vi "Dashboard Main.vi"() -> ()   [LabVIEW 2017]
uses:
  <vilib>/Utility/miscctls.llb/LVRowAndColumnTypeDef.ctl
  <vilib>/event_ctls.llb/eventvkey.ctl
  <vilib>/Rock Robotics/WPI/Dashboard/WPI_DashboardLogging Global.vi
panel:
  in  "Camera Settings Right":T1={"Frame Rate"=30, "Compression"=30, "Size"=1, "DB Camera Config"=FALSE} {"Frame Rate" scale=1.0..30.0; "Compression" scale=100.0..-1.0; "Size" items=["640x480", "320x240", "160x120"]}
  in  "Camera Name Right":string(combo)="No Camera Selection"
  out "Camera Info":cluster{"Mbps LED":bool, "Mbps":dbl, "fps":dbl} {"fps" format="%#.1g"; "Mbps" format="%#.1g"}
  in  "Camera Settings":T1={"Frame Rate"=30, "Compression"=30, "Size"=1, "DB Camera Config"=FALSE} {"Frame Rate" scale=1.0..30.0; "Compression" scale=100.0..-1.0; "Size" items=["640x480", "320x240", "160x120"]}
  in  "TCP":refnum<k5>
  in  "Rec Mode":enum32{"Stop", "Record", "Playback"}(radio)
  out "Robot IP":string
  out "Image Message":string="Timeout in Camera Communications"
  in  "Dashboard Tab":T2(tab)
  out "PowerCube Loaded":bool
  in  "Si Right":bool
  in  "Select Auto":string(combo)="Select Autonomous ..."
  out "NT Connection":bool
  out "Gyro":dbl(knob) scale=0.0..360.0
  out "Mode":T3(ring)=enum."Auto Disabled"
  out "Boolean":bool
  out "Boolean 2":bool
  out "Boolean 3":bool
  out "Boolean 4":bool
  out "Boolean 5":bool
  out "Boolean 6":bool
  out "Camera Image Right":T4(plugin-control)
  in  "DB/String 9":string
  in  "DB/String 8":string
  in  "DB/String 7":string
  in  "DB/String 6":string
  in  "DB/String 5":string
  in  "DB/String 4":string
  in  "DB/String 3":string
  in  "DB/String 2":string
  in  "DB/String 1":string
  in  "DB/String 0":string
  in  "DB/Slider 0":dbl(slide) scale=0.0..5.0
  in  "DB/Slider 1":dbl(slide) scale=0.0..5.0
  in  "DB/Slider 2":dbl(slide) scale=0.0..5.0
  in  "DB/Slider 3":dbl(slide) scale=0.0..5.0
  out "DB/LED 3":bool
  out "DB/LED 2":bool
  out "DB/LED 1":bool
  out "DB/LED 0":bool
  in  "DB/Button 3":bool
  in  "DB/Button 2":bool
  in  "DB/Button 1":bool
  in  "DB/Button 0":bool caption="New Name"
  out "Alliance":string
  out "GameData":string
  in  "Test Slider":dbl(slide) scale=0.0..100.0 scale format="%#_3g"
  in  "On/Off":bool caption="Solenoid"
  in  "Test Name":u16(ring) items=["Select the test to run..."]
  in  "Test Tree":string(tree)
  in  "Motor":cluster{"Value":dbl, "Enable":bool} {"Value" scale=-1.0..1.0 scale format="%#_3g"}
  out "Progress":T5 {"Test Progress" scale=0.0..100.0}
  in  "Rev/Fwd":cluster{"Forward":bool, "Reverse":bool}
  in  "Test Ring":u16(ring) items=["Monochrome", "Color"]
  out "Cmd Status":string
  in  "Execute Command":bool
  in  "Command Params":string[][](table)
  in  "Command Selection":i32(listbox)
  in  "CheckList":i32(listbox)
  out "Tree":string(tree)
  out "Camera Image":T4(plugin-control)
  out "Background":bool
  in  "Camera Name":string(combo)="No Camera Selection"
  # "HW"
  # "HW"
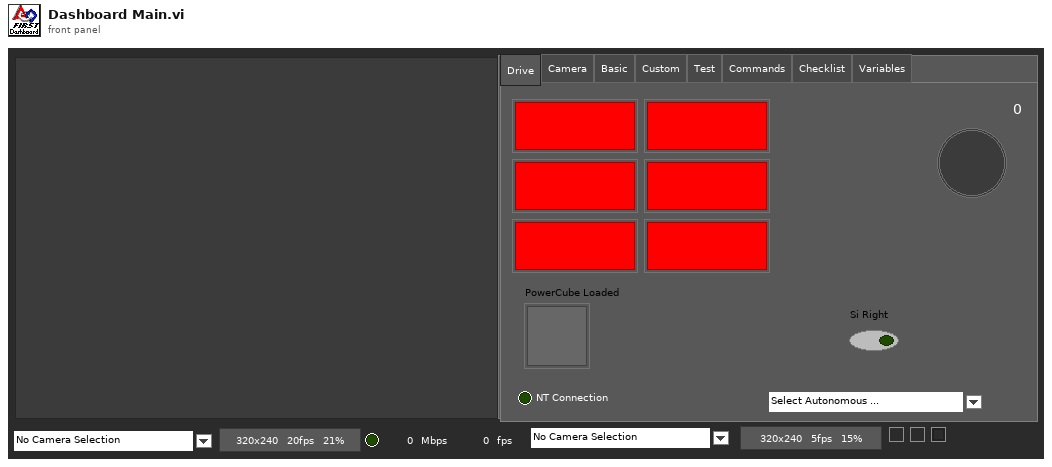
[diagram p1: front panel]
types:
  T1 = cluster{"Frame Rate":i32, "Compression":i32, "Size":u16, "DB Camera Config":bool}
  T2 = enum32{"Drive", "Camera", "Basic", "Custom", "Test", "Commands", "Checklist", "Variables"}
  T3 = enum8{"Tele-Op Disabled", "Tele-Op Enabled", "Auto Disabled", "Auto Enabled", "Test Disabled", "Test Enabled", "Disconnected", "No Code", "E-Stop"}
  T4 = typedef "IMAQ Image.ctl" = refnum<image>
  T5 = cluster{"Test Progress":u8, "Test Progress Text":string}
  T6 = cluster{"Save Path":path, "Interval (s)":dbl, "Keep":i32}
  T7 = typedef "Image Type" = u32
  T8 = cluster{"IDs":cluster{"RPC field ID":u16, "Unique ID":u16}, "String":string}
  T9 = cluster{"Error Strings":string, "Disable Counts":cluster{u16, u16}, "Rail Faults":cluster{u16, u16, u16}, "Robot IP":string, "DB Mode":u8, "Event Info":cluster{"Name":string, "Type":u8, "Number":u16, "Replay":u8}}
  T10 = cluster{"Storage":cluster{"Disk Free":u64, "RAM Block":u32, "RAM free":u32}, "CPU Utilization":cluster{"CPU % ISR":sgl, "CPU % Time Crit":sgl, "CPU % Timed Str":sgl, "CPU % High":sgl, "CPU % Above":sgl, "CPU % Normal":sgl, "CPU % Low":sgl}, "CAN":cluster{"% Bus Utilization":sgl, "Bus Off Cnt":u32, "TX_FIFO Full Cnt":u32, "Receive Error Cnt":u8, "Transmit Error Cnt":u8}, "HID":cluster{"HID Outputs":u32, "Rumble Low":u16, "Rumble High":u16}[]}
  T11 = cluster{"Status bits":cluster{"Test Mode":bool, "Autonomous":bool, "Enabled":bool, "Code Start":bool, "Brownout":bool, "Reserved 2":bool, "Reserved 3":bool, "E-Stop":bool}, "Code Trace":cluster{"Disabled":bool, "TeleOp":bool, "Auto":bool, "Test":bool}, "Controller Type":enum16{"unknown", "cRIO", "roboRio"}, "Code?":enum16{"unknown", "noCode", "code"}, "Battery V":dbl}
  T12 = cluster{"Control Bits":cluster{"TestMode":bool, "Autonomous":bool, "Enabled":bool, "FMS Present":bool, bool, bool, bool, "E-Stop":bool}, "Team Station ":u8, "Countdown":sgl, "Joystick Values":cluster{"Axes":dbl[], "Buttons":bool[], "POVs":i16[]}[]}
  T13 = cluster{"Axes":dbl[], "Buttons":bool[], "POVs":i16[]}[]
  T14 = cluster{"Axes":dbl[], "Buttons":bool[], "POVs":i16[]}
  T15 = cluster{"Camera Image":refnum<vi>, "Dashboard Tab":refnum<vi>, "Background":refnum<vi>, "Rec Mode":refnum<vi>, "Test Slider":refnum<vi>, "On/Off ":refnum<vi>, "Test Ring":refnum<vi>, "Rev/Fwd":refnum<vi>, "Test Name":refnum<vi>, "Motor":refnum<vi>, "Progress":refnum<vi>, "CheckList":refnum<vi>, "Tree":refnum<vi>, "Test Tree":refnum<vi>, "Command Params":refnum<vi>, "Command Selection":refnum<vi>, "Execute Command":refnum<vi>, "Cmd Status":refnum<vi>, "Camera Settings":refnum<vi>, "Camera Name":refnum<vi>, "Camera Info":refnum<vi>, "Camera Settings Right":refnum<vi>, "Camera Name Right":refnum<vi>, "Camera Image Right":refnum<vi>}
  T16 = cluster{"Camera Name":string, string, "Saved DB Images Info":cluster{"Save Path":path, "Interval (s)":dbl, "Keep":i32}}
  T17 = cluster{"Camera Name Right":string, string, "Saved DB Images Info":cluster{"Save Path":path, "Interval (s)":dbl, "Keep":i32}}
  T18 = cluster{"Operation":enum16{"Update", "Clear"}, "Color Box":u32}[]
  T19 = typedef "eventvkey.ctl" = enum16{"ASCII", "Enter", "Return", "Shift", "Ctrl", "Alt", "Cmd", "Opt", "Caps", "NumLock", "Clear", "Break", "Up", "Down", "Left", "Right", "Insert", "Delete", "Home", "End", "PageUp", "PageDown", "Escape", "Help", "Pause", "ScrollLock", "F1", "F2", "F3", "F4", "F5", "F6", "F7", "F8", "F9", "F10", "F11", "F12", "F13", "F14", "F15", "F16", "F17", "F18", "F19", "F20", "F21", "F22", "F23", "F24", "Play", "VolumeUp", "VolumeDown", "Mute", "Two Byte Char"}
  T20 = cluster{"Image Size":bool, "Image Type":bool, "Pixel Value":bool, "ROI Information":bool, "Zoom Factor":bool}
  T21 = cluster{"Operation":enum16{"Update", "Clear"}, "Color Box":u32}
  T22 = typedef "LVRowAndColumnTypeDef.ctl" = cluster{"Row":i32, "Column":i32}
  T23 = cluster{"Shift":bool, "Ctrl":bool, "Alt":bool, "Cmd":bool, "Opt":bool}
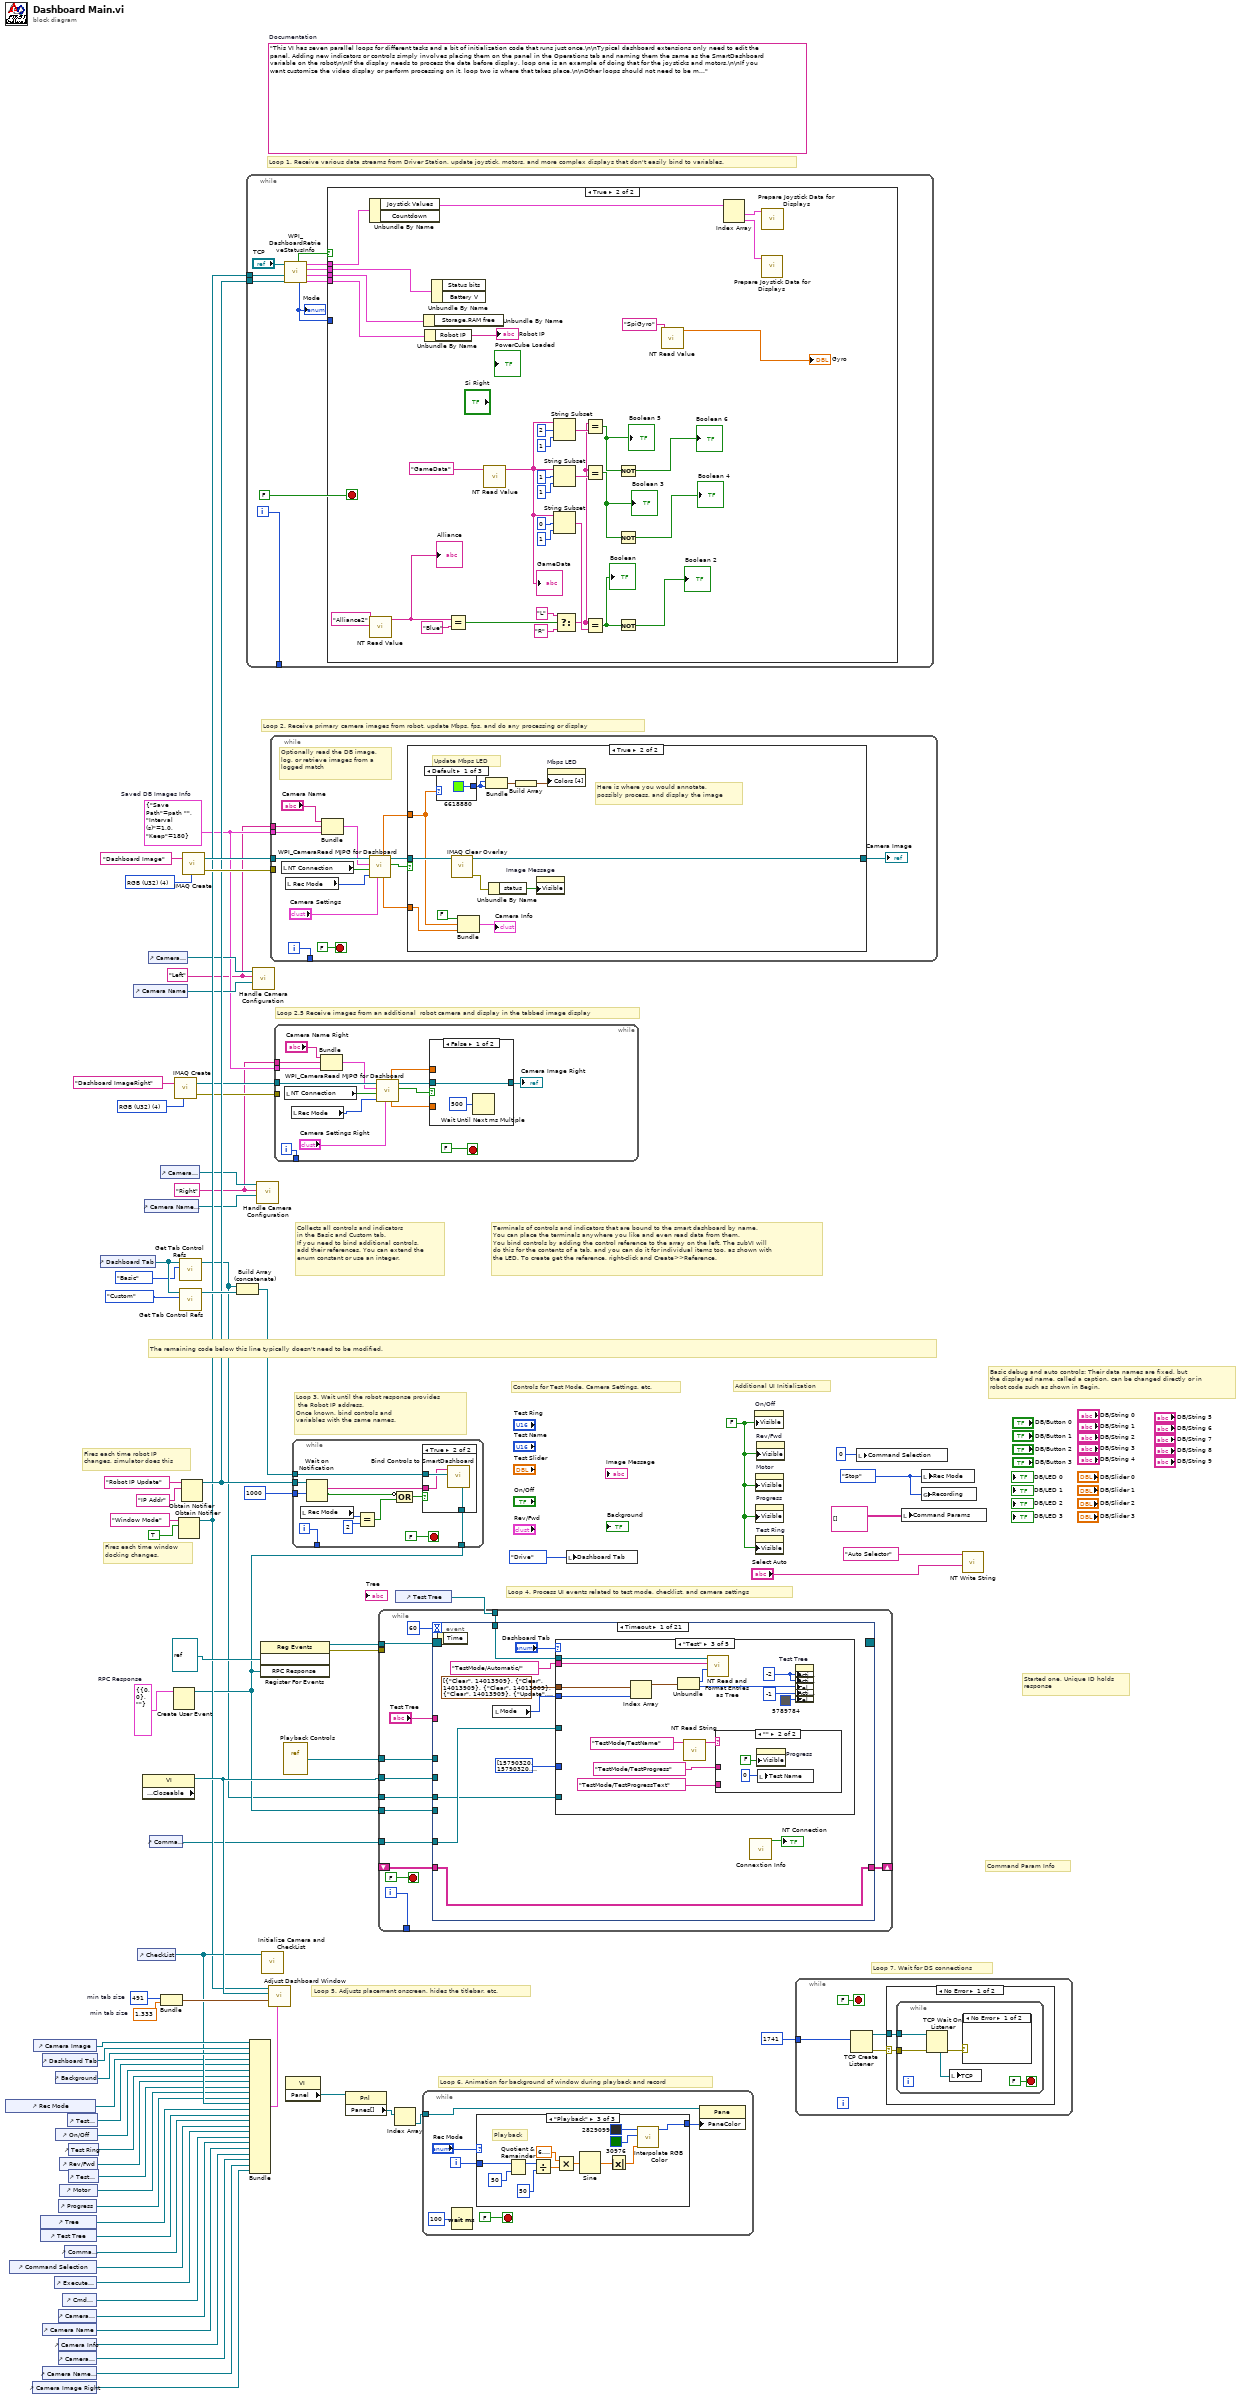
[diagram p0: block diagram]
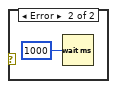
[diagram p3: hidden frame]
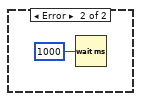
[diagram p4: hidden frame]
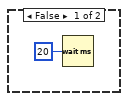
[diagram p5: hidden frame]
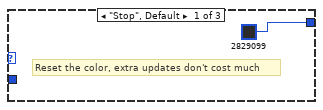
[diagram p6: hidden frame]
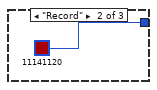
[diagram p7: hidden frame]
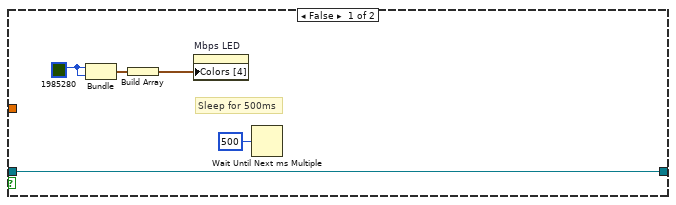
[diagram p9: hidden frame]
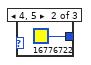
[diagram p10: hidden frame]
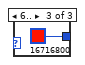
[diagram p11: hidden frame]
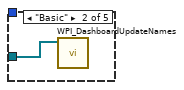
[diagram p13: hidden frame]
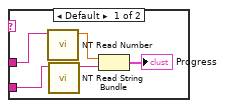
[diagram p14: hidden frame]
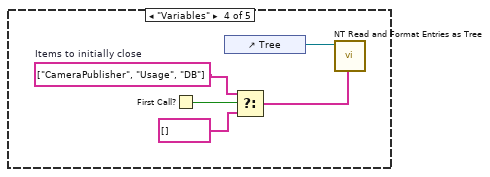
[diagram p15: hidden frame]
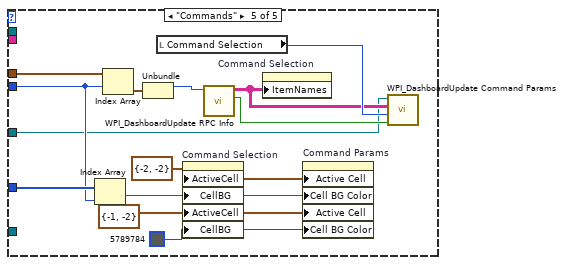
[diagram p16: hidden frame]
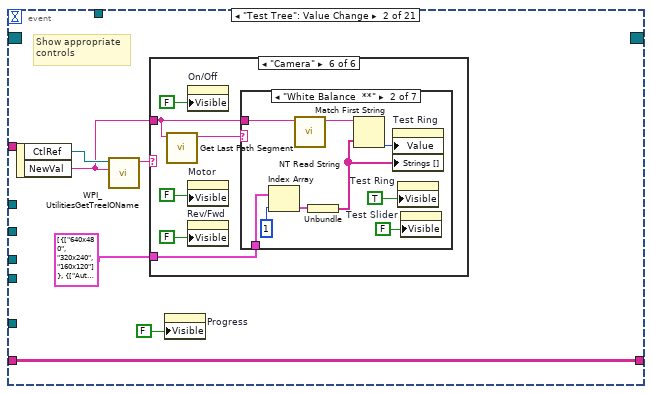
[diagram p17: hidden frame]
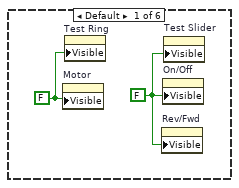
[diagram p18: hidden frame]
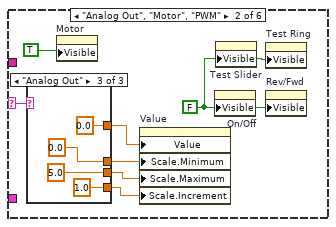
[diagram p19: hidden frame]
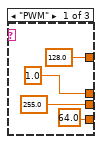
[diagram p20: hidden frame]
diagram:
  w3 = T6 {"Save Path"=path "", "Interval (s)"=1.0, "Keep"=180}  # Saved DB Images Info
  w2 = "Right"
  w1 = "Left"
  w13 = T7 4 items=["Grayscale (U8)", "Grayscale (I16)", "Grayscale (SGL)", "Complex (CSG)", "RGB (U32)", "HSL (U32)", "RGB (U64)"] ("Image Type")
  w29 = T8 {"IDs"={"RPC field ID"=0, "Unique ID"=0}, "String"=""}  # RPC Response
  w52 = 491  # min tab size
  w51 = 1.333  # min tab size
  w59 = enum32{"Stop", "Record", "Playback"}."Stop" ("Rec Mode")
  w36 = FALSE ("Visible")
  (unwired) "This VI has seven parallel loops for different tasks and a bit of initialization code that runs just once.\n\nTypical dashboard extensions only need to edit the panel. Adding new indicators or controls simply involves placing them on the panel in the Operations tab and naming them the same as the SmartDashboard variable on the robot\n\nIf the display needs to process the data before display, loop one is an example of doing that for the joysticks and motors.\n\nIf you want customize the video display or perform processing on it, loop two is where that takes place.\n\nOther loops should not need to be modified. They are pretty standard, and document the task they perform."  # Documentation
  w76 = T7 4 items=["Grayscale (U8)", "Grayscale (I16)", "Grayscale (SGL)", "Complex (CSG)", "RGB (U32)", "HSL (U32)", "RGB (U64)"] ("Image Type")
  # "Loop 2.5 Receive images from an additional  robot camera and display in the tabbed image display"
  # "Command Param Info"
  # "Started one, Unique ID holds\nresponse"
  # "Loop 7. Wait for DS connections"
  # "Basic debug and auto controls: Their data names are fixed, but\nthe displayed name, called a caption, can be changed directly or in\nrobot code such as shown in Begin."
  # "Controls for Test Mode, Camera Settings, etc."
  # "Additional UI Initialization"
  # "Loop 6. Animation for background of window during playback and record"
  # "Fires each time robot IP\nchanges, simulator does this"
  # "Fires each time window\ndocking changes."
  # "Collects all controls and indicators\nin the Basic and Custom tab.\nIf you need to bind additional controls,\nadd their references. You can extend the\nenum constant or use an integer."
  # "The remaining code below this line typically doesn't need to be modified."
  # "Loop 4. Process UI events related to test mode, checklist, and camera settings"
  # "Terminals of controls and indicators that are bound to the smart dashboard by name.\nYou can place the terminals anywhere you like and even read data from them.\nYou bind controls by adding the control reference to the array on the left. The subVI will\ndo this for the contents of a tab, and you can do it for individual items too, as shown with\nthe LED. To create get the reference, right-click and Create>>Reference."
  # "Loop 3. Wait until the robot response provides\n the Robot IP address.\nOnce known, bind controls and\nvariables with the same names."
  # "Loop 5. Adjusts placement onscreen, hides the titlebar, etc."
  # "Loop 1. Receive various data streams from Driver Station, update joystick, motors, and more complex displays that don't easily bind to variables."
  # "Loop 2. Receive primary camera images from robot, update Mbps, fps, and do any processing or display"
  n1 = control-ref of="Rec Mode"() -> (w42:refnum<vi>)
  n2 = control-ref of="Command Selection"() -> (w28:refnum<vi>)
  n3 = control-ref of="Camera Image Right"() -> (w6:refnum<vi>)
  n4 = control-ref of="Camera Image"() -> (w54:refnum<vi>)
  n5 = control-ref of="Tree"() -> (w46:refnum<vi>)
  n6 = control-ref of="Test Tree"() -> (w45:refnum<vi>)
  n7 = control-ref of="Dashboard Tab"() -> (w53:refnum<vi>)
  n8 = control-ref of="Camera Name"() -> (w19:refnum<vi>)
  n9 = control-ref of="Camera Name Right"() -> (w7:refnum<vi>)
  n10 = control-ref of="Execute Command"() -> (w30:refnum<vi>)
  n11 = control-ref of="Background"() -> (w49:refnum<vi>)
  n12 = control-ref of="On/Off"() -> (w40:refnum<vi>)
  n13 = control-ref of="Progress"() -> (w37:refnum<vi>)
  n14 = control-ref of="Camera Settings"() -> (w20:refnum<vi>)
  n15 = control-ref of="Camera Info"() -> (w18:refnum<vi>)
  n16 = control-ref of="Camera Settings Right"() -> (w8:refnum<vi>)
  n17 = control-ref of="Rev/Fwd"() -> (w38:refnum<vi>)
  n18 = control-ref of="Motor"() -> (w43:refnum<vi>)
  n19 = control-ref of="Cmd Status"() -> (w24:refnum<vi>)
  n20 = control-ref of="Command Params"() -> (w31:refnum<vi>)
  n21 = control-ref of="Test Slider"() -> (w41:refnum<vi>)
  n22 = control-ref of="Test Ring"() -> (w39:refnum<vi>)
  n23 = control-ref of="Test Name"() -> (w44:refnum<vi>)
  n24 = control-ref of="Dashboard Tab"() -> (w57:refnum<vi>)
  n25 = control-ref of="Camera Name"() -> (w21:refnum<vi>)
  n26 = control-ref of="CheckList"() -> (w47:refnum<vi>)
  n27 = property class="VI" props=["Front Panel.Closeable"]() -> (reference out=w58:refnum<vi>)  [unwired: 2 in, 2 out]
  n28 = control-ref of="Camera Name Right"() -> (w9:refnum<vi>)
  n29 = control-ref of="Camera Settings"() -> (w22:refnum<vi>)
  n30 = control-ref of="Command Params"() -> (w23:refnum<vi>)
  n31 = control-ref of="Camera Settings Right"() -> (w10:refnum<vi>)
  n32 = Bundle("min tab size"=w52, "min tab size"=w51) -> (w50:cluster{"min tab size":i32, "min tab size":dbl})  [unwired: 1 in]
  n33 = Create User Event(user event datatype=w29) -> (user event=w25:refnum<user-event>)  [unwired: 1 in, 1 out]
  n34 = call "IMAQ Create"("Image Name"="Dashboard ImageRight", "Image Type"=w13) -> ("New Image"=w12:T4, "error out"=w11:errorcluster)  [unwired: 2 in, 1 out]
  n35 = Obtain Notifier(name (unnamed)="Window Mode", notification data type=TRUE) -> (notifier out=w34:refnum<notifier>)  [unwired: 2 in, 2 out]
  n36 = call <vilib>:"Get Tab Control Refs.vi"("Page Index"=T2."Basic" ("Dashboard Tab"), "TabControl in"=w57) -> ("ControlsOnPage"=w17:refnum<vi>[])  [unwired: 9 in]
  n37 = call <vilib>:"Get Tab Control Refs.vi"("Page Index"=T2."Custom" ("Dashboard Tab"), "TabControl in"=w57) -> ("ControlsOnPage"=w56:refnum<vi>[])  [unwired: 9 in]
  n38 = Obtain Notifier(name (unnamed)="Robot IP Update", notification data type="IP Addr" ("name (unnamed)")) -> (notifier out=w35:refnum<notifier>)  [unwired: 2 in, 2 out]
  n39 = call "IMAQ Create"("Image Name"="Dashboard Image", "Image Type"=w76) -> ("New Image"=w74:T4, "error out"=w73:errorcluster)  [unwired: 2 in, 1 out]
  n40 = Build Array (concatenate)(w17, w56) -> (w55:refnum<vi>[])
  n41 = while {
    tunnel: [w86] -> _
    tunnel: w35 -> [w80]
    tunnel: w34 -> [w77]
    i -> [w86]
    stop <- FALSE stop-if-true
    n42 = call <vilib>:"WPI_DashboardRetrieveStatusInfo.vi"("Binding Refnum"=w80, "Window Mode Notifier"=w77, "TCP Cnx"="TCP") -> ("Power and Errors"=w81:T9, "Robot Metrics"=w84:T10, "Status Info"=w85:T11, "Control Info"=w82:T12, "Robot Mode"=w79:T3, "Process?"=w83:bool)  [unwired: 3 in]
    "Mode" <- w79
    n43 = case shown="True" w83 {
      tunnel: w85 -> [_ w122]
      tunnel: w84 -> [_ w121]
      tunnel: w82 -> [_ w120]
      tunnel: w81 -> [_ w119]
      tunnel: w79 -> [_ _]
      frame False {
        n44 = Wait (ms)(milliseconds to wait=u32 20) -> ()  [unwired: 1 out]
      }
      frame True {
        n45 = Unbundle By Name(w120) -> ("Joystick Values"=w118:T13)  [unwired: 1 out]
        n46 = call-poly <vilib>:"NT Read Value.vi"("Name"="Alliance2") -> ("String"=w91:string)  [unwired: 9 in, 1 out]
        "Alliance" <- w91
        n47 = Unbundle By Name(w121) -> ()  [unwired: 1 out]
        n48 = Unbundle By Name(w119) -> ("Robot IP"=→"Robot IP":string)
        n49 = Unbundle By Name(w122) -> ()  [unwired: 2 out]
        n50 = Equal?(x=w91, y="Blue") -> (x = y?=w112:bool)
        n51 = call-poly <vilib>:"NT Read Value.vi"("Name"="GameData") -> ("String"=w96:string)  [unwired: 9 in, 1 out]
        "GameData" <- w96
        n52 = String Subset(string=w96, offset (0)=2, length (rest)=1 ("length (rest)")) -> (substring=w113:string)
        n53 = String Subset(string=w96, offset (0)=1, length (rest)=1 ("length (rest)")) -> (substring=w115:string)
        n54 = String Subset(string=w96, offset (0)=0, length (rest)=1 ("length (rest)")) -> (substring=w114:string)
        n55 = Select(t="L" ("refnum name"), s=w112, f="R" ("refnum name")) -> (s? t:f=w97:string)
        n56 = Equal?(x=w97, y=w113) -> (x = y?=w99:bool)
        "Boolean 5" <- w99
        n57 = Equal?(x=w97, y=w115) -> (x = y?=w100:bool)
        "Boolean 3" <- w100
        n58 = Equal?(x=w97, y=w114) -> (x = y?=w103:bool)
        "Boolean" <- w103
        n59 = Not(x=w99) -> (.not. x?=→"Boolean 6":bool)
        n60 = Not(x=w100) -> (.not. x?=→"Boolean 4":bool)
        n61 = Not(x=w103) -> (.not. x?=→"Boolean 2":bool)
        n62 = call-poly <vilib>:"NT Read Value.vi"("Name"="SpiGyro") -> ("Numeric"=→"Gyro":dbl)  [unwired: 9 in, 1 out]
        n63 = Index Array(array=w118) -> (element #1=w117:T14, element #2=w116:T14)  [unwired: 2 in]
        n64 = call "Prepare Joystick Data for Displays.vi"("Joystick Values"=w116) -> ()  [unwired: 8 in, 3 out]
        n65 = call "Prepare Joystick Data for Displays.vi"("Joystick Values"=w117) -> ()  [unwired: 8 in, 3 out]
      }
    }
  }
  n66 = Bundle("Camera Image"=w54, "Dashboard Tab"=w53, "Background"=w49, "Rec Mode"=w42, "Test Slider"=w41, "On/Off"=w40, "Test Ring"=w39, "Rev/Fwd"=w38, "Test Name"=w44, "Motor"=w43, "Progress"=w37, "CheckList"=w47, "Tree"=w46, "Test Tree"=w45, "Command Params"=w31, "Command Selection"=w28, "Execute Command"=w30, "Cmd Status"=w24, "Camera Settings"=w20, "Camera Name"=w19, "Camera Info"=w18, "Camera Settings Right"=w8, "Camera Name Right"=w7, "Camera Image Right"=w6) -> (w48:T15)  [unwired: 1 in]
  n67 = call "Handle Camera Configuration.vi"("CameraNameRef"=w21, "Display Name"=w1, "ClusterRef"=w22) -> ()  [unwired: 9 in]
  n68 = call "Handle Camera Configuration.vi"("CameraNameRef"=w9, "Display Name"=w2, "ClusterRef"=w10) -> ()  [unwired: 9 in]
  n69 = register-events(refnum<vi> refnum, w25) -> (reference out=w63:refnum<event-registration>, error out=w62:errorcluster)  [unwired: 2 in]
  n70 = call "Initialize Camera and CheckList.vi"("ListBox in"=w47) -> ()  [unwired: 11 in]
  n71 = call "Adjust Dashboard Window.vi"("Sizing Refnums"=w48, "Size Constraints"=w50, "VI"=w58, "WIn Mode"=w34) -> ()  [unwired: 8 in]
  n72 = while {
    tunnel: w74 -> [w135]
    tunnel: w73 -> [_]
    tunnel: [w136] -> _
    tunnel: w3 -> [w126]
    tunnel: w1 -> [w123]
    i -> [w136]
    stop <- FALSE stop-if-true
    # "Optionally read the DB image,\nlog, or retrieve images from a\nlogged match"
    n73 = local read "NT Connection"() -> (w127:bool)
    n74 = local read "Rec Mode"() -> (w131:enum32{"Stop", "Record", "Playback"})
    n75 = Bundle("Camera Name"="Camera Name", w123, "Saved DB Images Info"=w126) -> (w125:T16)  [unwired: 1 in]
    n76 = call <vilib>:"WPI_CameraRead MJPG for Dashboard.vi"("Camera Settings"="Camera Settings", "Rec Mode"=w131, "NT Connection"=w127, "Capture Info"=w125, "Refnum in"=w135) -> ("Active"=w133:bool, "Refnum out"=w134:T4, "FPS"=w132:dbl, "Bandwidth (Mbps)"=w130:dbl)  [unwired: 3 in]
    n77 = case shown="True" w133 {
      tunnel: w134 -> [w138 w149]
      tunnel: w130 -> [_ w146]
      tunnel: w132 -> [_ w147]
      tunnel: [w138 w143] -> w128
      frame False {
        w140 = u32 1985280 ("Color Box")
        # "Sleep for 500ms"
        n78 = Bundle("Color Box"=w140, "Color Box"=w140) -> (w141:cluster{"Color Box":u32, "Color Box":u32})  [unwired: 1 out]
        n79 = Build Array(w141) -> (w139:cluster{"Color Box":u32, "Color Box":u32}[])
        n80 = property on="Mbps LED" class="Bool (strict)"("Colors [4]"=w139) -> ()  [unwired: 2 in, 2 out]
        n81 = Wait Until Next ms Multiple(millisecond multiple=u32 500) -> ()  [unwired: 1 out]
      }
      frame True {
        # "Here is where you would annotate,\npossibly process, and display the image"
        # "Update Mbps LED"
        n82 = case shown="Default" w146 {
          tunnel: [u32 6618880 ("Color Box") u32 16776722 ("Color Box") u32 16716800 ("Color Box")] -> w150
          frame Default {
          }
          frame 4, 5 {
          }
          frame 6.. {
          }
        }
        n83 = call "IMAQ Clear Overlay"("Image"=w149) -> ("error out"=w152:errorcluster, "Image Out"=w143:T4)  [unwired: 2 in, 7 out]
        n84 = Bundle(FALSE, "Bandwidth (Mbps)"=w146, "FPS"=w147) -> (→"Camera Info":cluster{bool, "Bandwidth (Mbps)":dbl, "FPS":dbl})  [unwired: 1 in]
        n85 = Bundle("Color Box"=w150, "Color Box"=w150) -> (w151:cluster{"Color Box":u32, "Color Box":u32})  [unwired: 1 out]
        n86 = Unbundle By Name(w152) -> ("status"=w153:bool)
        n87 = Build Array(w151) -> (w148:cluster{"Color Box":u32, "Color Box":u32}[])
        n88 = property on="Image Message" class="Str"("Visible"=w153) -> ()  [unwired: 2 in, 2 out]
        n89 = property on="Mbps LED" class="Bool (strict)"("Colors [4]"=w148) -> ()  [unwired: 2 in, 2 out]
      }
    }
    "Camera Image" <- w128
  }
  n90 = while {
    tunnel: w12 -> [w171]
    tunnel: w11 -> [_]
    tunnel: [w166] -> _
    tunnel: w3 -> [w160]
    tunnel: w2 -> [w157]
    i -> [w166]
    stop <- FALSE stop-if-true
    n91 = local read "NT Connection"() -> (w161:bool)
    n92 = local read "Rec Mode"() -> (w170:enum32{"Stop", "Record", "Playback"})
    n93 = Bundle("Camera Name Right"="Camera Name Right", w157, "Saved DB Images Info"=w160) -> (w159:T17)  [unwired: 1 in]
    n94 = call <vilib>:"WPI_CameraRead MJPG for Dashboard.vi"("Camera Settings"="Camera Settings Right", "Rec Mode"=w170, "NT Connection"=w161, "Capture Info"=w159, "Refnum in"=w171) -> ("Active"=w165:bool, "Refnum out"=w168:T4, "FPS"=w163:dbl, "Bandwidth (Mbps)"=w164:dbl)  [unwired: 3 in]
    n95 = case shown="False" w165 {
      tunnel: w168 -> [w172 w174]
      tunnel: w164 -> [_ _]
      tunnel: w163 -> [_ _]
      tunnel: [w172 w174] -> w162
      frame False {
        n96 = Wait Until Next ms Multiple(millisecond multiple=u32 500) -> ()  [unwired: 1 out]
      }
      frame True {
      }
    }
    "Camera Image Right" <- w162
  }
  n97 = vi-ref "Playback Controls.vi"() -> (w64:refnum<vi>)
  n98 = property class="VI"() -> ("Panel"=w66:refnum<vi>)  [unwired: 2 in, 2 out]
  n99 = while {
    tunnel: w55 -> [w186]
    tunnel: w35 -> [w184]
    tunnel: [w182] -> _
    tunnel: u32 1000 ("milliseconds to wait") -> [w181]
    tunnel: w25 -> [w175]
    i -> [w182]
    stop <- FALSE stop-if-true
    n100 = local read "Rec Mode"() -> (w177:enum32{"Stop", "Record", "Playback"})
    n101 = Wait on Notification(notifier=w184, timeout in ms (-1)=w181) -> (notification=w183:string, timed out?=w179:bool)  [unwired: 2 in, 2 out]
    n102 = Equal?(x=w177, y=u16 2 ("Rec Mode")) -> (x = y?=w178:bool)
    n103 = Compound Arithmetic op=OR(invert w179, w178) -> (w180:bool)
    n104 = case shown="True" w180 {
      tunnel: w186 -> [_ w189]
      tunnel: w183 -> [_ w188]
      tunnel: w175 -> [_ w187]
      frame False {
      }
      frame True {
        n105 = call <vilib>:"Bind Controls to SmartDashboard.vi"("RPC ref"=w187, "Bound Control Refs"=w189, "Server IP Address"=w188) -> ()  [unwired: 9 in]
      }
    }
  }
  n106 = property class="Pnl"(reference=w66) -> ("Panes[]"=w67:refnum<vi>[])  [unwired: 1 in, 2 out]
  n107 = Index Array(array=w67) -> (element=w65:refnum<vi>)  [unwired: 1 in]
  n108 = control-ref of="Test Tree"() -> (w68:refnum<vi>)
  n109 = while {
    tunnel: [w199] -> _
    tunnel: w68 -> [w198]
    tunnel: w64 -> [w197]
    tunnel: w63 -> [w196]
    tunnel: w62 -> [_]
    tunnel: w58 -> [w195]
    tunnel: w25 -> [w194]
    tunnel: w23 -> [w193]
    shift-right: [w192] -> _
    shift-left: _ -> [w191]
    tunnel: w17 -> [w190]
    i -> [w199]
    stop <- FALSE stop-if-true
    n110 = event shown="[0] Timeout" {
      selector: w196 -> [_ _ _ _ _ _ _ _ _ _ _ _ _ _ _ _ _ _ _ _ _]
      dyn-events: [_ _ _ _ _ _ _ _ _ _ _ _ _ _ _ _ w459 _ _ _ _] -> _
      timeout: u32 60 ("milliseconds to wait") -> [_ _ _ _ _ _ _ _ _ _ _ _ _ _ _ _ _ _ _ _ _]
      tunnel: w198 -> [w211 _ _ _ _ _ _ _ _ _ _ _ _ _ _ _ _ _ _ _ _]
      tunnel: "Test Tree" -> [_ _ _ _ _ _ _ _ _ _ _ w426 w434 w436 w440 w448 _ _ _ _ _]
      tunnel: w197 -> [_ _ _ _ _ _ _ _ _ _ _ _ _ _ _ _ w461 _ w479 _ _]
      tunnel: w195 -> [_ _ _ _ _ _ _ _ _ _ _ _ _ _ _ _ w457 _ _ _ _]
      tunnel: w194 -> [_ _ _ _ _ _ _ _ _ _ _ _ _ _ _ _ w455 _ _ _ _]
      tunnel: w193 -> [w206 _ _ _ _ _ w377 _ _ _ _ _ _ _ _ _ _ _ _ _ _]
      tunnel: [w205 w254 w356 w361 w370 w374 w375 w384 w394 w401 w413 w425 w432 w435 w439 w447 w454 w474 w476 w480 w493] -> w192
      tunnel: w191 -> [w205 w254 w356 w361 w370 w374 w375 _ _ w401 w413 w425 w432 w435 w439 w447 w454 w474 w476 w480 w493]
      tunnel: w190 -> [w203 _ _ _ _ _ _ _ _ _ _ _ _ _ _ _ _ _ _ _ _]
      event Timeout {
        n111 = event-data() -> ()  [unwired: 1 in, 1 out]
        n112 = local read "Mode"() -> (w208:T3)
        n113 = case shown="\"Test\"" "Dashboard Tab" {
          tunnel: w211 -> [_ _ w227 _ _]
          tunnel: "TestMode/Automatic/" ("Name Pattern") -> [_ _ w226 _ _]
          tunnel: T18 [{"Operation"=enum."Clear", "Color Box"=14013909}, {"Operation"=enum."Clear", "Color Box"=14013909}, {"Operation"=enum."Clear", "Color Box"=14013909}, {"Operation"=enum."Clear", "Color Box"=14013909}, {"Operation"=enum."Update", "Color Box"=14013909}, {"Operation"=enum."Update", "Color Box"=16777215}, {"Operation"=enum."Clear", "Color Box"=14013909}, {"Operation"=enum."Clear", "Color Box"=14013909}, {"Operation"=enum."Clear", "Color Box"=14013909}] -> [_ _ w219 _ w247]
          tunnel: w208 -> [_ _ w218 _ w246]
          tunnel: u32[] [15790320, 15790320, 15790320, 15790320, 16777215, 16777215, 15790320, 15790320, 15790320] -> [_ _ _ _ w252]
          tunnel: w206 -> [_ _ _ _ w240]
          tunnel: w203 -> [_ w213 _ _ _]
          frame "Custom", Default {
          }
          frame "Basic" {
            n114 = call <vilib>:"WPI_DashboardUpdateNames.vi"("Controls on Tab"=w213) -> ()  [unwired: 11 in]
          }
          frame "Test" {
            w225 = -2 ("Active Item:Row Number")
            n115 = Index Array(array=w219, index=w218) -> (element=w220:T21)
            n116 = Unbundle(w220) -> ("Operation"=w221:enum16{"Update", "Clear"}, "Color Box"=w222:u32)
            n117 = call <vilib>:"NT Read String.vi"("Name"="TestMode/TestName") -> ("String"=w216:string)  [unwired: 9 in, 1 out]
            n118 = call <vilib>:"NT Read and Format Entries as Tree.vi"("Operation"=w221, "Name Pattern"=w226, "Tree Refnum"=w227) -> ()  [unwired: 7 in, 2 out]
            n119 = case shown="\"\"" w216 {
              tunnel: "TestMode/TestProgress" ("Name") -> [w229 _]
              tunnel: "TestMode/TestProgressText" ("Name") -> [w228 _]
              frame Default {
                n120 = call <vilib>:"NT Read Number.vi"("Name"=w229) -> ("Numeric"=w230:dbl)  [unwired: 9 in, 1 out]
                n121 = call <vilib>:"NT Read String.vi"("Name"=w228) -> ("String"=w231:string)  [unwired: 9 in, 1 out]
                n122 = Bundle("Numeric"=w230, "String"=w231) -> (→"Progress":cluster{"Numeric":dbl, "String":string})  [unwired: 1 in]
              }
              frame "" {
                n123 = property on="Progress" class="Clust (strict)"("Visible"=FALSE) -> ()  [unwired: 2 in, 2 out]
                n124 = local write "Test Name"(u16 0) -> ()
              }
            }
            n125 = property on="Test Tree" class="Tree (strict)"("Active Item Row Number"=w225, "ActiveColNum"=w225, "CellBG"=w222, "Active Item Row Number"=-1 ("Active Item:Row Number"), "CellBG"=u32 5789784 ("Color Box")) -> ()  [unwired: 2 in, 2 out]
          }
          frame "Variables" {
            w237 = string[] ["CameraPublisher", "Usage", "DB"]  # Items to initially close
            n126 = First Call?() -> (First Call?: T/F=w238:bool)
            n127 = control-ref of="Tree"() -> (w239:refnum<vi>)
            n128 = Select(t=w237, s=w238, f=string[] []) -> (s? t:f=w235:string[])
            n129 = call <vilib>:"NT Read and Format Entries as Tree.vi"("Tags to  Close"=w235, "Tree Refnum"=w239) -> ()  [unwired: 8 in, 2 out]
          }
          frame "Commands" {
            w248 = u32 5789784 ("Color Box")
            w249 = T22 {"Row"=-1, "Column"=-2} ("Active Cell:Active Cell")
            w251 = T22 {"Row"=-2, "Column"=-2} ("Active Cell:Active Cell")
            n130 = Index Array(array=w252, index=w246) -> (element=w250:u32)
            n131 = Index Array(array=w247, index=w246) -> (element=w245:T21)
            n132 = Unbundle(w245) -> ("Operation"=w244:enum16{"Update", "Clear"})  [unwired: 1 out]
            n133 = local read "Command Selection"() -> (w243:i32)
            n134 = property on="Command Selection" class="MCListbox (strict)"("ActiveCell"=w251, "CellBG"=w250, "ActiveCell"=w249, "CellBG"=w248) -> ()  [unwired: 2 in, 2 out]
            n135 = call <vilib>:"WPI_DashboardUpdate RPC Info.vi"("Operation"=w244) -> ("update"=w242:bool, "commands"=w241:string[][])  [unwired: 9 in]
            n136 = property on="Command Selection" class="MCListbox (strict)"("ItemNames"=w241) -> ()  [unwired: 2 in, 2 out]
            n137 = property on="Command Params" class="Tbl (strict)"("Active Cell"=w251, "Cell BG Color"=w250, "Active Cell"=w249, "Cell BG Color"=w248) -> ()  [unwired: 2 in, 2 out]
            n138 = call <vilib>:"WPI_DashboardUpdate Command Params.vi"("Update"=w242, "NewVal"=w243, "Commands"=w241, "Param Tbl"=w240) -> ()  [unwired: 7 in, 1 out]
          }
        }
        n139 = call <vilib>:"Connextion Info.vi"() -> ("Connected"=→"NT Connection":bool)  [unwired: 10 in, 1 out]
      }
      event "Test Tree": Value Change {
        # "Show appropriate\ncontrols"
        n140 = event-data() -> ("CtlRef"=w257:refnum<vi>, "NewVal"=w255:string)  [unwired: 1 in]
        n141 = call <vilib>:"WPI_UtilitiesGetTreeIOName.vi"("NewVal"=w255, "TreeControl in"=w257) -> ("I/O Name"=w258:string)  [unwired: 9 in]
        n142 = case shown="\"Camera\"" w258 {
          selector: w258 -> [_ w265 _ w287 w296 _]
          tunnel: w255 -> [_ _ w284 w286 _ w303]
          tunnel: cluster{string[]}[] [{["640x480", "320x240", "160x120"]}, {["Auto", "Fixed indoor", "Fixed outdoor 1", "Fixed outdoor 2", "Fixed fluorescent 1", "Fixed fluorescent 2", "Hold current"]}, {["Auto", "Flicker-free 50 Hz", "Flicker-free 60 Hz", "Hold current"]}, {["None", "Prioritize frame rate", "Prioritize image quality"]}, {["Monochrome", "Color"]}] -> [_ _ _ _ _ w302]
          frame Default {
            w260 = FALSE ("Visible")
            w259 = FALSE ("Visible")
            n143 = property on="Motor" class="Clust (strict)"("Visible"=w259) -> ()  [unwired: 2 in, 2 out]
            n144 = property on="Test Ring" class="Ring (strict)"("Visible"=w259) -> ()  [unwired: 2 in, 2 out]
            n145 = property on="Rev/Fwd" class="Clust (strict)"("Visible"=w260) -> ()  [unwired: 2 in, 2 out]
            n146 = property on="On/Off" class="Bool (strict)"("Visible"=w260) -> ()  [unwired: 2 in, 2 out]
            n147 = property on="Test Slider" class="Slide (strict)"("Visible"=w260) -> ()  [unwired: 2 in, 2 out]
          }
          frame "Analog Out", "Motor", "PWM" {
            w266 = FALSE ("Visible")
            n148 = case shown="\"Analog Out\"" w265 {
              tunnel: [1.0 ("Value") -1.0 ("Value") 0.0 ("Value")] -> w264
              tunnel: [255.0 ("Value") 1.0 ("Value") 5.0 ("Value")] -> w263
              tunnel: [128.0 ("Value") 0.0 ("Value") 0.0 ("Value")] -> w262
              tunnel: [64.0 ("Value") 0.5 ("Value") 1.0 ("Value")] -> w261
              frame "PWM" {
              }
              frame "Motor", Default {
              }
              frame "Analog Out" {
              }
            }
            n149 = property on="Motor" class="Clust (strict)"("Visible"=TRUE) -> ()  [unwired: 2 in, 2 out]
            n150 = property on="Value" class="Slide (strict)"("Value"=w262, "Scale.Minimum"=w264, "Scale.Maximum"=w263, "Scale.Increment"=w261) -> ()  [unwired: 2 in, 2 out]
            n151 = property on="On/Off" class="Bool (strict)"("Visible"=w266) -> ()  [unwired: 2 in, 2 out]
            n152 = property on="Test Slider" class="Slide (strict)"("Visible"=w266) -> ()  [unwired: 2 in, 2 out]
            n153 = property on="Test Ring" class="Ring (strict)"("Visible"=w266) -> ()  [unwired: 2 in, 2 out]
            n154 = property on="Rev/Fwd" class="Clust (strict)"("Visible"=w266) -> ()  [unwired: 2 in, 2 out]
          }
          frame "Servo" {
            w282 = FALSE ("Visible")
            n155 = call <vilib>:"NT Read Number.vi"("Name"=w284) -> ("Numeric"=w283:dbl)  [unwired: 9 in, 1 out]
            n156 = property on="Test Slider" class="Slide (strict)"("Visible"=TRUE, "Scale.Maximum"=170.0 ("Scale.Range:Maximum")) -> ()  [unwired: 2 in, 2 out]
            n157 = local write "Test Slider"(w283) -> ()
            n158 = property on="Motor" class="Clust (strict)"("Visible"=w282) -> ()  [unwired: 2 in, 2 out]
            n159 = property on="Rev/Fwd" class="Clust (strict)"("Visible"=w282) -> ()  [unwired: 2 in, 2 out]
            n160 = property on="On/Off" class="Bool (strict)"("Visible"=w282) -> ()  [unwired: 2 in, 2 out]
            n161 = property on="Test Ring" class="Ring (strict)"("Visible"=w282) -> ()  [unwired: 2 in, 2 out]
          }
          frame "Relay", "Solenoid" {
            w285 = FALSE ("Visible")
            n162 = property on="Motor" class="Clust (strict)"("Visible"=w285) -> ()  [unwired: 2 in, 2 out]
            n163 = property on="Test Slider" class="Slide (strict)"("Visible"=w285) -> ()  [unwired: 2 in, 2 out]
            n164 = Search and Replace String(input string=w286, search string="/Value  **", replace string="/Direction") -> (result string=w292:string)  [unwired: 5 in, 3 out]
            n165 = property on="Test Ring" class="Ring (strict)"("Visible"=w285) -> ()  [unwired: 2 in, 2 out]
            n166 = call <vilib>:"NT Read String.vi"("Name"=w292) -> ("String"=w290:string)  [unwired: 9 in, 1 out]
            n167 = Equal?(x="Both directions", y=w290) -> (x = y?=w288:bool)
            n168 = Not(x=w288) -> (.not. x?=w289:bool)
            n169 = property on="Rev/Fwd" class="Clust (strict)"("Visible"=w288) -> ()  [unwired: 2 in, 2 out]
            n170 = property on="On/Off" class="Bool (strict)"("Visible"=w289, "Caption.Text"=w287) -> ()  [unwired: 2 in, 2 out]
          }
          frame "Compressor", "Digital Out" {
            w295 = FALSE ("Visible")
            # "Get direction and finish"
            n171 = property on="Motor" class="Clust (strict)"("Visible"=w295) -> ()  [unwired: 2 in, 2 out]
            n172 = property on="Test Slider" class="Slide (strict)"("Visible"=w295) -> ()  [unwired: 2 in, 2 out]
            n173 = property on="Test Ring" class="Ring (strict)"("Visible"=w295) -> ()  [unwired: 2 in, 2 out]
            n174 = property on="On/Off" class="Bool (strict)"("Visible"=TRUE, "Caption.Text"=w296) -> ()  [unwired: 2 in, 2 out]
            n175 = property on="Rev/Fwd" class="Clust (strict)"("Visible"=FALSE) -> ()  [unwired: 2 in, 2 out]
          }
          frame "Camera" {
            n176 = call <vilib>:"Get Last Path Segment.vi"("String in"=w303) -> ("String out"=w304:string)  [unwired: 10 in]
            n177 = property on="On/Off" class="Bool (strict)"("Visible"=FALSE) -> ()  [unwired: 2 in, 2 out]
            n178 = property on="Motor" class="Clust (strict)"("Visible"=FALSE) -> ()  [unwired: 2 in, 2 out]
            n179 = property on="Rev/Fwd" class="Clust (strict)"("Visible"=FALSE) -> ()  [unwired: 2 in, 2 out]
            n180 = case shown="\"White Balance  **\"" w304 {
              tunnel: w303 -> [w310 w319 w328 w337 w346 _ w352]
              tunnel: w302 -> [w308 w316 w325 w334 w343 _ _]
              frame "Size  **" {
                n181 = Index Array(array=w308) -> (element=w307:cluster{string[]})  [unwired: 1 in]
                n182 = call <vilib>:"NT Read String.vi"("Name"=w310) -> ("String"=w309:string)  [unwired: 9 in, 1 out]
                n183 = Unbundle(w307) -> (w305:string[])
                n184 = Match First String(2:w305, 3:w309) -> (0:w306:i32)  [unwired: 1 out]
                n185 = property on="Test Ring" class="Ring (strict)"("Value"=w306, "Strings []"=w305) -> ()  [unwired: 2 in, 2 out]
                n186 = property on="Test Ring" class="Ring (strict)"("Visible"=TRUE) -> ()  [unwired: 2 in, 2 out]
                n187 = property on="Test Slider" class="Slide (strict)"("Visible"=FALSE) -> ()  [unwired: 2 in, 2 out]
              }
              frame "White Balance  **" {
                n188 = Index Array(array=w316, index=1) -> (element=w317:cluster{string[]})
                n189 = call <vilib>:"NT Read String.vi"("Name"=w319) -> ("String"=w318:string)  [unwired: 9 in, 1 out]
                n190 = Unbundle(w317) -> (w314:string[])
                n191 = Match First String(2:w314, 3:w318) -> (0:w313:i32)  [unwired: 1 out]
                n192 = property on="Test Ring" class="Ring (strict)"("Value"=w313, "Strings []"=w314) -> ()  [unwired: 2 in, 2 out]
                n193 = property on="Test Ring" class="Ring (strict)"("Visible"=TRUE) -> ()  [unwired: 2 in, 2 out]
                n194 = property on="Test Slider" class="Slide (strict)"("Visible"=FALSE) -> ()  [unwired: 2 in, 2 out]
              }
              frame "Exposure  **" {
                n195 = Index Array(array=w325, index=2) -> (element=w326:cluster{string[]})
                n196 = call <vilib>:"NT Read String.vi"("Name"=w328) -> ("String"=w327:string)  [unwired: 9 in, 1 out]
                n197 = Unbundle(w326) -> (w322:string[])
                n198 = Match First String(2:w322, 3:w327) -> (0:w323:i32)  [unwired: 1 out]
                n199 = property on="Test Ring" class="Ring (strict)"("Value"=w323, "Strings []"=w322) -> ()  [unwired: 2 in, 2 out]
                n200 = property on="Test Ring" class="Ring (strict)"("Visible"=TRUE) -> ()  [unwired: 2 in, 2 out]
                n201 = property on="Test Slider" class="Slide (strict)"("Visible"=FALSE) -> ()  [unwired: 2 in, 2 out]
              }
              frame "Exposure Priority  **" {
                n202 = Index Array(array=w334, index=3) -> (element=w335:cluster{string[]})
                n203 = call <vilib>:"NT Read String.vi"("Name"=w337) -> ("String"=w336:string)  [unwired: 9 in, 1 out]
                n204 = Unbundle(w335) -> (w331:string[])
                n205 = Match First String(2:w331, 3:w336) -> (0:w332:i32)  [unwired: 1 out]
                n206 = property on="Test Ring" class="Ring (strict)"("Value"=w332, "Strings []"=w331) -> ()  [unwired: 2 in, 2 out]
                n207 = property on="Test Ring" class="Ring (strict)"("Visible"=TRUE) -> ()  [unwired: 2 in, 2 out]
                n208 = property on="Test Slider" class="Slide (strict)"("Visible"=FALSE) -> ()  [unwired: 2 in, 2 out]
              }
              frame "Color Enable  **" {
                n209 = Index Array(array=w343, index=4) -> (element=w344:cluster{string[]})
                n210 = call <vilib>:"NT Read String.vi"("Name"=w346) -> ("String"=w345:string)  [unwired: 9 in, 1 out]
                n211 = Unbundle(w344) -> (w340:string[])
                n212 = Match First String(2:w340, 3:w345) -> (0:w341:i32)  [unwired: 1 out]
                n213 = property on="Test Ring" class="Ring (strict)"("Value"=w341, "Strings []"=w340) -> ()  [unwired: 2 in, 2 out]
                n214 = property on="Test Ring" class="Ring (strict)"("Visible"=TRUE) -> ()  [unwired: 2 in, 2 out]
                n215 = property on="Test Slider" class="Slide (strict)"("Visible"=FALSE) -> ()  [unwired: 2 in, 2 out]
              }
              frame Default {
                n216 = property on="Test Ring" class="Ring (strict)"("Visible"=FALSE) -> ()  [unwired: 2 in, 2 out]
                n217 = property on="Test Slider" class="Slide (strict)"("Visible"=FALSE) -> ()  [unwired: 2 in, 2 out]
              }
              frame "Brightness  **", "Color Level  **", "Compression  **", "FPS  **", "Sharpness  **" {
                n218 = call <vilib>:"NT Read Number.vi"("Name"=w352) -> ("Numeric"=w351:dbl)  [unwired: 9 in, 1 out]
                n219 = local write "Test Slider"(w351) -> ()
                n220 = property on="Test Slider" class="Slide (strict)"("Visible"=TRUE, "Scale.Maximum"=100.0 ("Scale.Range:Maximum")) -> ()  [unwired: 2 in, 2 out]
                n221 = property on="Test Ring" class="Ring (strict)"("Visible"=FALSE) -> ()  [unwired: 2 in, 2 out]
              }
            }
          }
        }
        n222 = property on="Progress" class="Clust (strict)"("Visible"=FALSE) -> ()  [unwired: 2 in, 2 out]
      }
      event "Test Name": Mouse Enter {
        # "Populate the ring with the list of tests"
        n223 = event-data() -> ()  [unwired: 1 in, 1 out]
        n224 = call <vilib>:"NT Read String Array.vi"("Name"="TestMode/TestList") -> ("String Array"=w360:string[])  [unwired: 9 in, 1 out]
        n225 = Build Array (concatenate)("Select the test to run...", w360) -> (w359:string[])
        n226 = property on="Test Name" class="Ring (strict)"("Strings []"=w359) -> ()  [unwired: 2 in, 2 out]
      }
      event "Test Name": Value Change {
        w362 = FALSE ("Visible")
        # "Tell the robot the test name to run"
        n227 = event-data() -> ("NewVal"=w366:u16)  [unwired: 1 in]
        n228 = property on="Test Name" class="Ring (strict)"() -> ("Strings []"=w367:string[])  [unwired: 2 in, 2 out]
        n229 = local write "Progress"(T5 {"Test Progress"=0, "Test Progress Text"=""} ("Progress")) -> ()
        n230 = Index Array(array=w367, index=w366) -> (element=w365:string)
        n231 = call <vilib>:"NT Write String.vi"("String"=w365, "Name"="TestMode/TestName") -> ()  [unwired: 9 in, 1 out]
        n232 = property on="Progress" class="Clust (strict)"("Visible"=TRUE) -> ()  [unwired: 2 in, 2 out]
        n233 = property on="Motor" class="Clust (strict)"("Visible"=w362) -> ()  [unwired: 2 in, 2 out]
        n234 = property on="Test Slider" class="Slide (strict)"("Visible"=w362) -> ()  [unwired: 2 in, 2 out]
        n235 = property on="On/Off" class="Bool (strict)"("Visible"=w362) -> ()  [unwired: 2 in, 2 out]
        n236 = property on="Rev/Fwd" class="Clust (strict)"("Visible"=w362) -> ()  [unwired: 2 in, 2 out]
        n237 = property on="Test Ring" class="Ring (strict)"("Visible"=w362) -> ()  [unwired: 2 in, 2 out]
      }
      event "Select Auto": Mouse Enter {
        # "Populate the combo box with the list of autonomous options"
        n238 = event-data() -> ()  [unwired: 1 in, 1 out]
        n239 = call <vilib>:"NT Read String Array.vi"("Name"="Auto List") -> ("String Array"=w369:string[])  [unwired: 9 in, 1 out]
        n240 = property on="Select Auto" class="CmbBox"("Strings[]"=w369) -> ()  [unwired: 2 in, 2 out]
      }
      event "Select Auto": Value Change {
        # "User modified the Auto Selection. Write to NT variable so robot knows."
        n241 = event-data() -> ("NewVal"=w372:string)  [unwired: 1 in]
        n242 = call <vilib>:"NT Write String.vi"("String"=w372, "Name"="Auto Selector") -> ()  [unwired: 9 in, 1 out]
      }
      event "Command Selection": Value Change {
        # "Get the params and show in table"
        n243 = event-data() -> ("NewVal"=w378:i32)  [unwired: 1 in]
        n244 = property on="Command Selection" class="MCListbox (strict)"() -> ("ItemNames"=w376:string[][])  [unwired: 2 in, 2 out]
        n245 = call <vilib>:"WPI_DashboardUpdate Command Params.vi"("NewVal"=w378, "Commands"=w376, "Param Tbl"=w377) -> ()  [unwired: 8 in, 1 out]
      }
      event "Execute Command": Value Change {
        # "Started one, Unique ID holds\nresponse"
        n246 = event-data() -> ()  [unwired: 1 in, 1 out]
        n247 = property on="Command Selection" class="MCListbox (strict)"() -> ("ItemNames"=w389:string[][])  [unwired: 2 in, 2 out]
        n248 = Index Array(array=w389, index (row)="Command Selection", index (col)=0) -> (element=w387:string)
        n249 = call <vilib>:"Invoke Commands.vi"("Command Params"="Command Params", "Function Name"=w387) -> ("Params"=w383:u8, "Started"=w382:bool)  [unwired: 7 in, 1 out]
        n250 = Array Subset(array="Command Params", length (row)=w383) -> (w384:string[][])  [unwired: 3 in]
        n251 = Select(t="Executing" ("Cmd Status"), s=w382, f="" ("Cmd Status")) -> (s? t:f=→"Cmd Status":string)
      }
      event "Command Selection": Double Click {
        n252 = event-data() -> ("Row"=w397:i32)  [unwired: 1 in]
        n253 = property on="Command Selection" class="MCListbox (strict)"() -> ("ItemNames"=w400:string[][])  [unwired: 2 in, 2 out]
        n254 = local read "Command Params"() -> (w396:string[][])
        n255 = Index Array(array=w400, index (row)=w397, index (col)=0) -> (element=w398:string)
        n256 = call <vilib>:"Invoke Commands.vi"("Command Params"=w396, "Function Name"=w398) -> ("Params"=w395:u8, "Started"=w390:bool)  [unwired: 7 in, 1 out]
        n257 = Array Subset(array=w396, length (row)=w395) -> (w394:string[][])  [unwired: 3 in]
        n258 = Select(t="Executing" ("Cmd Status"), s=w390, f="" ("Cmd Status")) -> (s? t:f=w391:string)
        n259 = local write "Cmd Status"(w391) -> ()
      }
      event "CheckList": Double Click {
        # "Shift clears all"
        # "Update symbols on the listbox"
        n260 = event-data() -> ("PlatMods.Shift"=w402:bool, "Row"=w404:i32)  [unwired: 1 in]
        n261 = case shown="True" w402 {
          tunnel: w404 -> [w408 _]
          tunnel: 1 -> [w407 _]
          frame False {
            n262 = property on="CheckList" class="LstBox (strict)"() -> ("Item Symbols"=w406:i32[])  [unwired: 2 in, 2 out]
            n263 = Replace Array Subset(array=w406, new element=w407, index=w408) -> (w405:i32[])
            n264 = property on="CheckList" class="LstBox (strict)"("Item Symbols"=w405) -> ()  [unwired: 2 in, 2 out]
          }
          frame True {
            w409 = 0 ("Top Row")
            n265 = property on="CheckList" class="LstBox (strict)"() -> ("Number of Rows"=w411:u32)  [unwired: 2 in, 2 out]
            n266 = Initialize Array(0, w411) -> (w410:i32[])
            n267 = property on="CheckList" class="LstBox (strict)"("Top Row"=w409, "Value"=w409, "Item Symbols"=w410) -> ()  [unwired: 2 in, 2 out]
          }
        }
      }
      event "CheckList": Key Down {
        # "Update symbols on the listbox\nLeft and right keys check and uncheck"
        n268 = event-data() -> ("VKey"=w415:T19)  [unwired: 1 in]
        n269 = case shown="\"Left\", \"Right\"" w415 {
          selector: w415 -> [w420 _]
          tunnel: eventvkey."Left" ("VKey") -> [w418 _]
          frame "Left", "Right" {
            n270 = Equal?(x=w418, y=w420) -> (x = y?=w419:bool)
            n271 = Select(t=0, s=w419, f=1) -> (s? t:f=w421:i32)
            n272 = property on="CheckList" class="LstBox (strict)"() -> ("Item Symbols"=w424:i32[])  [unwired: 2 in, 2 out]
            n273 = Replace Array Subset(array=w424, new element=w421, index="CheckList") -> (w423:i32[])
            n274 = property on="CheckList" class="LstBox (strict)"("Item Symbols"=w423) -> ()  [unwired: 2 in, 2 out]
          }
          frame Default {
          }
        }
      }
      event "Motor.Enable": Value Change {
        # "When the test mode otor enable helper is set, update that\ntree row item's value"
        n275 = event-data() -> ("NewVal"=w430:bool)  [unwired: 1 in]
        n276 = Unbundle("Motor") -> ("Value"=w429:dbl)  [unwired: 1 out]
        n277 = Select(t=w429, s=w430, f=0.0) -> (s? t:f=w427:dbl)
        n278 = call <vilib>:"NT Write Number.vi"("Numeric"=w427, "Name"=w426) -> ()  [unwired: 9 in, 1 out]
      }
      event "Test Slider": Value Change {
        # "When the test mode slider helper is set, update that\ntree row item's value"
        n279 = event-data() -> ("NewVal"=w433:dbl)  [unwired: 1 in]
        n280 = call <vilib>:"NT Write Number.vi"("Numeric"=w433, "Name"=w434) -> ()  [unwired: 9 in, 1 out]
      }
      event "On/Off": Value Change {
        # "When the test mode on/off helper value is set, update that\ntree row item's value"
        n281 = event-data() -> ("NewVal"=w438:bool)  [unwired: 1 in]
        n282 = Boolean To (0,1)(Boolean=w438) -> (0, 1=w437:i16)
        n283 = call <vilib>:"NT Write Number.vi"("Numeric"=w437, "Name"=w436) -> ()  [unwired: 9 in, 1 out]
      }
      event "Rev/Fwd": Value Change {
        # "When the test mode helper value for relays is set, update that\ntree row item's value"
        n284 = event-data() -> ("NewVal.Forward"=w446:bool, "NewVal.Reverse"=w445:bool)  [unwired: 1 in]
        n285 = Boolean To (0,1)(Boolean=w446) -> (0, 1=w442:i16)
        n286 = Boolean To (0,1)(Boolean=w445) -> (0, 1=w444:i16)
        n287 = Negate(x=w444) -> (-x=w443:i16)
        n288 = Add(x=w442, y=w443) -> (x+y=w441:i16)
        n289 = call <vilib>:"NT Write Number.vi"("Numeric"=w441, "Name"=w440) -> ()  [unwired: 9 in, 1 out]
      }
      event "Test Ring": Value Change {
        # "When a test mode helper value is selected from the ring,\nset the tree item's variable to the string value"
        n290 = event-data() -> ("NewVal"=w450:u16)  [unwired: 1 in]
        n291 = property on="Test Ring" class="Ring (strict)"() -> ("Strings []"=w451:string[])  [unwired: 2 in, 2 out]
        n292 = Index Array(array=w451, index=w450) -> (element=w449:string)
        n293 = call <vilib>:"NT Write String.vi"("String"=w449, "Name"=w448) -> ()  [unwired: 9 in, 1 out]
      }
      event "Rec Mode": Value Change {
        # "Update globals for recording mode and path to read log from.\nClear when logging and let NetworkTables set path for vision to\nuse."
        n294 = event-data() -> ("NewVal"=w462:enum32{"Stop", "Record", "Playback"})  [unwired: 1 in]
        n295 = global write "WPI_DashboardLogging Global.vi" "Logging Filename"(path "") -> ()
        n296 = global write "WPI_DashboardLogging Global.vi" "Recording"(w462) -> ()
        n297 = case shown="\"Playback\"" w462 {
          tunnel: w461 -> [_ w464 w473]
          tunnel: [_ _ w472] -> w459
          tunnel: [_ _ w471] -> _
          tunnel: w457 -> [_ _ w469]
          tunnel: cluster{i32, i32} {-250, 170} -> [_ _ w468]
          tunnel: [_ _ T20 {"Image Size"=TRUE, "Image Type"=TRUE, "Pixel Value"=TRUE, "ROI Information"=TRUE, "Zoom Factor"=FALSE} ("Image Information Shown:All Elements")] -> w452
          tunnel: [_ _ TRUE ("Zoom Factor")] -> w453
          tunnel: w455 -> [_ _ w465]
          frame Default {
          }
          frame "Stop", "Record" {
            # "Place Window too"
            n298 = invoke class="VI" method="FP.Close"(reference=w464) -> (reference out=w463:refnum<vi>)  [unwired: 2 in, 2 out]
            n299 = invoke class="VI" method="Abort VI"(reference=w463) -> ()  [unwired: 2 in, 3 out]
          }
          frame "Playback" {
            n300 = call "Open Playback Panel.vi"("Offset"=w468, "DB VI Ref"=w469, "Playback in"=w473) -> ("Playback out"=w470:refnum<vi>)  [unwired: 8 in]
            n301 = register-events(w470, w465) -> (reference out=w472:refnum<event-registration>, error out=w471:errorcluster)  [unwired: 2 in]
          }
        }
        n302 = property on="Camera Image Right" class="ImageControl"("Image Information Shown"=w452, "Image Information Visible"=w453) -> ()  [unwired: 2 in, 2 out]
        n303 = property on="Camera Image" class="ImageControl"("Image Information Shown"=w452, "Image Information Visible"=w453) -> ()  [unwired: 2 in, 2 out]
        n304 = call <vilib>:"WPI_DashboardNT Log FieldName Cache.vi"("Operation"=enum16{"Lookup/Add", "Index", "Clear"}."Clear") -> ()  [unwired: 8 in, 3 out]
      }
      event Panel Close {
        w475 = enum32{"Stop", "Record", "Playback"}."Stop" ("Rec Mode")
        # "Playback window has been closed, abort"
        n305 = event-data() -> ()  [unwired: 1 in, 4 out]
        n306 = local write "Rec Mode"(w475) -> ()
        n307 = global write "WPI_DashboardLogging Global.vi" "Recording"(w475) -> ()
      }
      event Panel Close {
        # "Abort playback window and ourself"
        n308 = event-data() -> ()  [unwired: 1 in, 4 out]
        n309 = invoke class="VI" method="FP.Close"(reference=w479) -> (reference out=w478:refnum<vi>)  [unwired: 2 in, 2 out]
        n310 = invoke class="VI" method="Abort VI"(reference=w478) -> (error out=w477:errorcluster)  [unwired: 2 in, 2 out]
        n311 = invoke class="VI" method="Abort VI"(error in=w477) -> ()  [unwired: 2 in, 3 out]
      }
      event User Event {
        n312 = event-data() -> ("IDs"=w486:cluster{"RPC field ID":u16, "Unique ID":u16}, "String"=w485:string)  [unwired: 1 in]
        n313 = Bundle("IDs"=w486, "String"=w485) -> (w484:T8)  [unwired: 1 in]
        n314 = call <vilib>:"Retrieve RPC Response.vi"("RPC Response"=w484) -> ("Output"=w482:string[][])  [unwired: 10 in]
        n315 = Build Array (concatenate)(w480, w482) -> (w481:string[][])
        n316 = local write "Command Params"(w481) -> ()
        n317 = local write "Cmd Status"("" ("Cmd Status")) -> ()
      }
      event "Tree": Double Click {
        n318 = event-data() -> ("PlatMods"=w492:T23, "Tag"=w489:string)  [unwired: 1 in]
        n319 = Unbundle(w492) -> ("Shift"=w491:bool)  [unwired: 4 out]
        n320 = String Subset(string=w489, length (rest)=1 ("length (rest)")) -> (substring=w488:string)  [unwired: 1 in]
        n321 = Not(x=w491) -> (.not. x?=w490:bool)
        n322 = case shown="\"/\"" w488 {
          tunnel: w489 -> [_ w495]
          tunnel: w490 -> [_ w494]
          frame Default {
          }
          frame "/" {
            n323 = call <vilib>:"NT Update Persistence.vi"("Persistence"=w494, "Name"=w495) -> ()  [unwired: 9 in, 1 out]
          }
        }
      }
    }
  }
  n324 = while {
    tunnel: w65 -> [w497]
    i -> [w500]
    stop <- FALSE stop-if-true
    n325 = Wait (ms)(milliseconds to wait=u32 100) -> ()  [unwired: 1 out]
    n326 = case shown="\"Playback\"" "Rec Mode" {
      tunnel: w500 -> [_ _ w515]
      tunnel: [u32 2829099 ("Base Color") u32 11141120 ("Target Color") w504] -> w496
      frame "Stop", Default {
        # "Reset the color, extra updates don't cost much"
      }
      frame "Record" {
      }
      frame "Playback" {
        # "Playback"
        n327 = Quotient & Remainder(x=w515, y=u32 50 ("milliseconds to wait")) -> (x-y*floor(x/y)=w511:u32)  [unwired: 1 out]
        n328 = Divide(x=w511, y=u32 50 ("milliseconds to wait")) -> (x/y=w508:dbl)
        n329 = Multiply(x=6.283185307179586, y=w508) -> (x*y=w513:dbl)
        n330 = Sine(x=w513) -> (sin(x)=w512:dbl)
        n331 = Absolute Value(x=w512) -> (abs(x)=w505:dbl)
        n332 = call "Interpolate RGB Color.vi"("Proportion"=w505, "Target Color"=u32 30976, "Base Color"=u32 2829099) -> ("Result Color"=w504:u32)  [unwired: 8 in]
      }
    }
    n333 = property class="Pane"(reference=w497, "PaneColor"=w496) -> ()  [unwired: 1 in, 2 out]
  }
  n334 = local write "Dashboard Tab"(T2."Drive" ("Dashboard Tab")) -> ()
  n335 = property on="On/Off" class="Bool (strict)"("Visible"=w36) -> ()  [unwired: 2 in, 2 out]
  n336 = property on="Motor" class="Clust (strict)"("Visible"=w36) -> ()  [unwired: 2 in, 2 out]
  n337 = property on="Progress" class="Clust (strict)"("Visible"=w36) -> ()  [unwired: 2 in, 2 out]
  n338 = property on="Test Ring" class="Ring (strict)"("Visible"=w36) -> ()  [unwired: 2 in, 2 out]
  n339 = property on="Rev/Fwd" class="Clust (strict)"("Visible"=w36) -> ()  [unwired: 2 in, 2 out]
  n340 = while {
    tunnel: u16 1741 ("timeout ms (25000)") -> [w517]
    stop <- FALSE stop-if-true
    n341 = TCP Create Listener(10:w517) -> (0:w516:errorcluster, 3:w518:refnum<k5>)  [unwired: 4 in, 1 out]
    n342 = case shown="No Error" w516 {
      selector: w516 -> [w520 _]
      tunnel: w518 -> [w521 _]
      frame No Error {
        n343 = while {
          tunnel: w521 -> [w524]
          tunnel: w520 -> [w523]
          stop <- FALSE stop-if-true
          n344 = TCP Wait On Listener(8:w523, 11:w524) -> (0:w525:errorcluster, 4:w526:refnum<k5>)  [unwired: 2 in, 3 out]
          n345 = local write "TCP"(w526) -> ()
          n346 = case shown="No Error" w525 {
            frame No Error {
            }
            frame Error {
              n347 = Wait (ms)(milliseconds to wait=u32 1000) -> ()  [unwired: 1 out]
            }
          }
        }
      }
      frame Error {
        n348 = Wait (ms)(milliseconds to wait=u32 1000) -> ()  [unwired: 1 out]
      }
    }
  }
  n349 = local write "Command Selection"(u16 0 ("milliseconds to wait")) -> ()
  n350 = local write "Command Params"(string[][] [] ("Command Params")) -> ()
  n351 = global write "WPI_DashboardLogging Global.vi" "Recording"(w59) -> ()
  n352 = local write "Rec Mode"(w59) -> ()
  n353 = call <vilib>:"NT Write String.vi"("String"="Select Auto", "Name"="Auto Selector") -> ()  [unwired: 9 in, 1 out]
